vi "Benchmark SV Receive LV2012 - NI Verified - 1000 Byte - 1Var.vi"() -> ()   [LabVIEW 2019]
uses:
  <vilib>/Platform/TimedLoop/XDataNode/timing_clust.ctl
  <vilib>/Platform/TimedLoop/XDataNode/nitl_modes.ctl
  <vilib>/Platform/TimedLoop/XDataNode/wakeup.ctl
  <vilib>/platform/TimedLoop/XDataNode/XDataNode.xnode
  <vilib>/Platform/TimedLoop/XDataNode/XDNodeRunTimeDep.lvlib
panel:
  out "output cluster 2":T1
  in  "stop":bool
  in  "Server Closed":string="The server VI closed the connection."
  out "Time":u32
  out "Counter":i32
  # "Overview:  Coding that exemplifies how to benchmark the communication of Shared Variables.\nRequirements: LabVIEW 2012 or compatible\nInstructions:\n1. Run this VI\n2. Watch the amount of time it takes to communicate on the \"Benchmark SV Send  LV2012 - NI Verified.vi\" \n3. Stop both VIs"
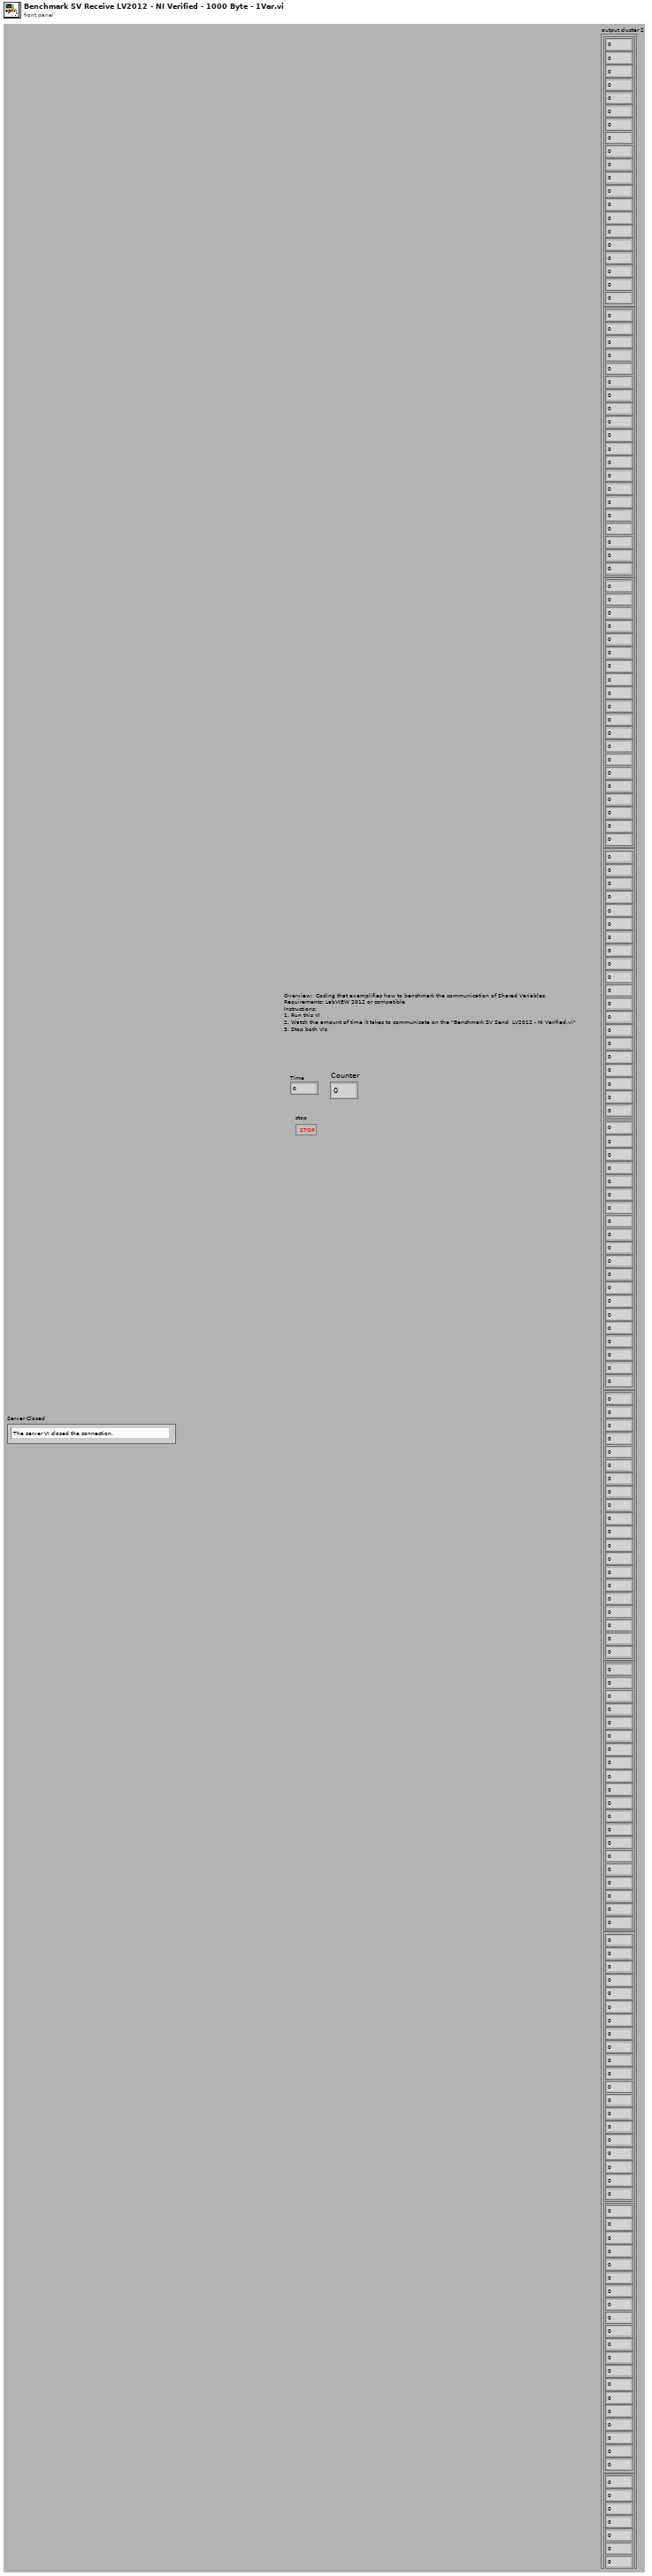
[diagram p1: front panel]
types:
  T1 = cluster{cluster{i64, i64, i64, i64, i64, i64, i64, i64, i64, i64, i64, i64, i64, i64, i64, i64, i64, i64, i64, i64}, cluster{i64, i64, i64, i64, i64, i64, i64, i64, i64, i64, i64, i64, i64, i64, i64, i64, i64, i64, i64, i64}, cluster{i64, i64, i64, i64, i64, i64, i64, i64, i64, i64, i64, i64, i64, i64, i64, i64, i64, i64, i64, i64}, cluster{i64, i64, i64, i64, i64, i64, i64, i64, i64, i64, i64, i64, i64, i64, i64, i64, i64, i64, i64, i64}, cluster{i64, i64, i64, i64, i64, i64, i64, i64, i64, i64, i64, i64, i64, i64, i64, i64, i64, i64, i64, i64}, cluster{i64, i64, i64, i64, i64, i64, i64, i64, i64, i64, i64, i64, i64, i64, i64, i64, i64, i64, i64, i64}, cluster{i64, i64, i64, i64, i64, i64, i64, i64, i64, i64, i64, i64, i64, i64, i64, i64, i64, i64, i64, i64}, cluster{i64, i64, i64, i64, i64, i64, i64, i64, i64, i64, i64, i64, i64, i64, i64, i64, i64, i64, i64, i64}, cluster{i64, i64, i64, i64, i64, i64, i64, i64, i64, i64, i64, i64, i64, i64, i64, i64, i64, i64, i64, i64}, cluster{i64, i64, i64, i64, i64, i64, i64, i64, i64, i64, i64, i64, i64, i64, i64, i64, i64, i64, i64, i64}, cluster{i64, i64, i64, i64, i64, i64, i64, i64, i64, i64, i64, i64, i64, i64, i64, i64, i64, i64, i64, i64}, cluster{i64, i64, i64, i64, i64, i64, i64, i64, i64, i64, i64, i64, i64, i64, i64, i64, i64, i64, i64, i64}, cluster{i64, i64, i64, i64, i64, i64, i64, i64, i64, i64, i64, i64, i64, i64, i64, i64, i64, i64, i64, i64}, cluster{i64, i64, i64, i64, i64, i64, i64, i64, i64, i64, i64, i64, i64, i64, i64, i64, i64, i64, i64, i64}, cluster{i64, i64, i64, i64, i64, i64, i64, i64, i64, i64, i64, i64, i64, i64, i64, i64, i64, i64, i64, i64}, cluster{i64, i64, i64, i64, i64, i64, i64, i64, i64, i64, i64, i64, i64, i64, i64, i64, i64, i64, i64, i64}, cluster{i64, i64, i64, i64, i64, i64, i64, i64, i64, i64, i64, i64, i64, i64, i64, i64, i64, i64, i64, i64}, cluster{i64, i64, i64, i64, i64, i64, i64, i64, i64, i64, i64, i64, i64, i64, i64, i64, i64, i64, i64, i64}, cluster{i64, i64, i64, i64, i64, i64, i64, i64, i64, i64, i64, i64, i64, i64, i64, i64, i64, i64, i64, i64}, cluster{i64, i64, i64, i64, i64, i64, i64, i64, i64, i64, i64, i64, i64, i64, i64, i64, i64, i64, i64, i64}, cluster{i64, i64, i64, i64, i64, i64, i64, i64, i64, i64, i64, i64, i64, i64, i64, i64, i64, i64, i64, i64}, cluster{i64, i64, i64, i64, i64, i64, i64, i64, i64, i64, i64, i64, i64, i64, i64, i64, i64, i64, i64, i64}, cluster{i64, i64, i64, i64, i64, i64, i64, i64, i64, i64, i64, i64, i64, i64, i64, i64, i64, i64, i64, i64}, cluster{i64, i64, i64, i64, i64, i64, i64, i64, i64, i64, i64, i64, i64, i64, i64, i64, i64, i64, i64, i64}, cluster{i64, i64, i64, i64, i64, i64, i64, i64, i64, i64, i64, i64, i64, i64, i64, i64, i64, i64, i64, i64}, cluster{i64, i64, i64, i64, i64, i64, i64, i64, i64, i64, i64, i64, i64, i64, i64, i64, i64, i64, i64, i64}, cluster{i64, i64, i64, i64, i64, i64, i64, i64, i64, i64, i64, i64, i64, i64, i64, i64, i64, i64, i64, i64}, cluster{i64, i64, i64, i64, i64, i64, i64, i64, i64, i64, i64, i64, i64, i64, i64, i64, i64, i64, i64, i64}, cluster{i64, i64, i64, i64, i64, i64, i64, i64, i64, i64, i64, i64, i64, i64, i64, i64, i64, i64, i64, i64}, cluster{i64, i64, i64, i64, i64, i64, i64, i64, i64, i64, i64, i64, i64, i64, i64, i64, i64, i64, i64, i64}, cluster{i64, i64, i64, i64, i64, i64, i64, i64, i64, i64, i64, i64, i64, i64, i64, i64, i64, i64, i64, i64}, cluster{i64, i64, i64, i64, i64, i64, i64, i64, i64, i64, i64, i64, i64, i64, i64, i64, i64, i64, i64, i64}, cluster{i64, i64, i64, i64, i64, i64, i64, i64, i64, i64, i64, i64, i64, i64, i64, i64, i64, i64, i64, i64}, cluster{i64, i64, i64, i64, i64, i64, i64, i64, i64, i64, i64, i64, i64, i64, i64, i64, i64, i64, i64, i64}, cluster{i64, i64, i64, i64, i64, i64, i64, i64, i64, i64, i64, i64, i64, i64, i64, i64, i64, i64, i64, i64}, cluster{i64, i64, i64, i64, i64, i64, i64, i64, i64, i64, i64, i64, i64, i64, i64, i64, i64, i64, i64, i64}, cluster{i64, i64, i64, i64, i64, i64, i64, i64, i64, i64, i64, i64, i64, i64, i64, i64, i64, i64, i64, i64}, cluster{i64, i64, i64, i64, i64, i64, i64, i64, i64, i64, i64, i64, i64, i64, i64, i64, i64, i64, i64, i64}, cluster{i64, i64, i64, i64, i64, i64, i64, i64, i64, i64, i64, i64, i64, i64, i64, i64, i64, i64, i64, i64}, cluster{i64, i64, i64, i64, i64, i64, i64, i64, i64, i64, i64, i64, i64, i64, i64, i64, i64, i64, i64, i64}, cluster{i64, i64, i64, i64, i64, i64, i64, i64, i64, i64, i64, i64, i64, i64, i64, i64, i64, i64, i64, i64}, cluster{i64, i64, i64, i64, i64, i64, i64, i64, i64, i64, i64, i64, i64, i64, i64, i64, i64, i64, i64, i64}, cluster{i64, i64, i64, i64, i64, i64, i64, i64, i64, i64, i64, i64, i64, i64, i64, i64, i64, i64, i64, i64}, cluster{i64, i64, i64, i64, i64, i64, i64, i64, i64, i64, i64, i64, i64, i64, i64, i64, i64, i64, i64, i64}, cluster{i64, i64, i64, i64, i64, i64, i64, i64, i64, i64, i64, i64, i64, i64, i64, i64, i64, i64, i64, i64}, cluster{i64, i64, i64, i64, i64, i64, i64, i64, i64, i64, i64, i64, i64, i64, i64, i64, i64, i64, i64, i64}, cluster{i64, i64, i64, i64, i64, i64, i64, i64, i64, i64, i64, i64, i64, i64, i64, i64, i64, i64, i64, i64}, cluster{i64, i64, i64, i64, i64, i64, i64, i64, i64, i64, i64, i64, i64, i64, i64, i64, i64, i64, i64, i64}, cluster{i64, i64, i64, i64, i64, i64, i64, i64, i64, i64, i64, i64, i64, i64, i64, i64, i64, i64, i64, i64}, cluster{i64, i64, i64, i64, i64, i64, i64, i64, i64, i64, i64, i64, i64, i64, i64, i64, i64, i64, i64, i64}}
  T2 = typedef "XDNodeRunTimeDep.lvlib/timing_clust.ctl" = cluster{"Expected End [f-1]":u64, "Actual End [f-1]":u64, "Finished Late? [f-1]":bool, "Expected End [i-1]":u64, "Actual End [i-1]":u64, "Finished Late? [i-1]":bool, "Expected Start [i]":u64, "Actual Start [i]":u64, "Expected Start [f]":u64, "Actual Start [f]":u64, "Source Name":string, "Structure Name":string, "Period":i64, "Deadline":i64, "Offset":i64, "Start":i64, "Priority":i32, "Timeout":i32, "Mode":T3, "Wakeup Reason":T4, "Error":errorcluster, "Source Type":string, "Secondary Source Type":string, "Global End Time":u64, "Global Start Time":u64, "Frame Duration":u64, "Iteration Duration":u64, "Assigned CPU":i32, "I/O Scan Engine Mode":u32}
  T3 = typedef "XDNodeRunTimeDep.lvlib/nitl_modes.ctl" = enum32{"No Change", "Process missed periods, maintain original phase", "Discard missed periods, maintain original phase", "Process missed periods, ignore original phase", "Discard missed periods, ignore original phase"}
  T4 = typedef "XDNodeRunTimeDep.lvlib/wakeup.ctl" = enum32{"Normal", "Aborted", "Asynchronous wakeup", "Timing source error", "Timed loop error", "Timeout"}
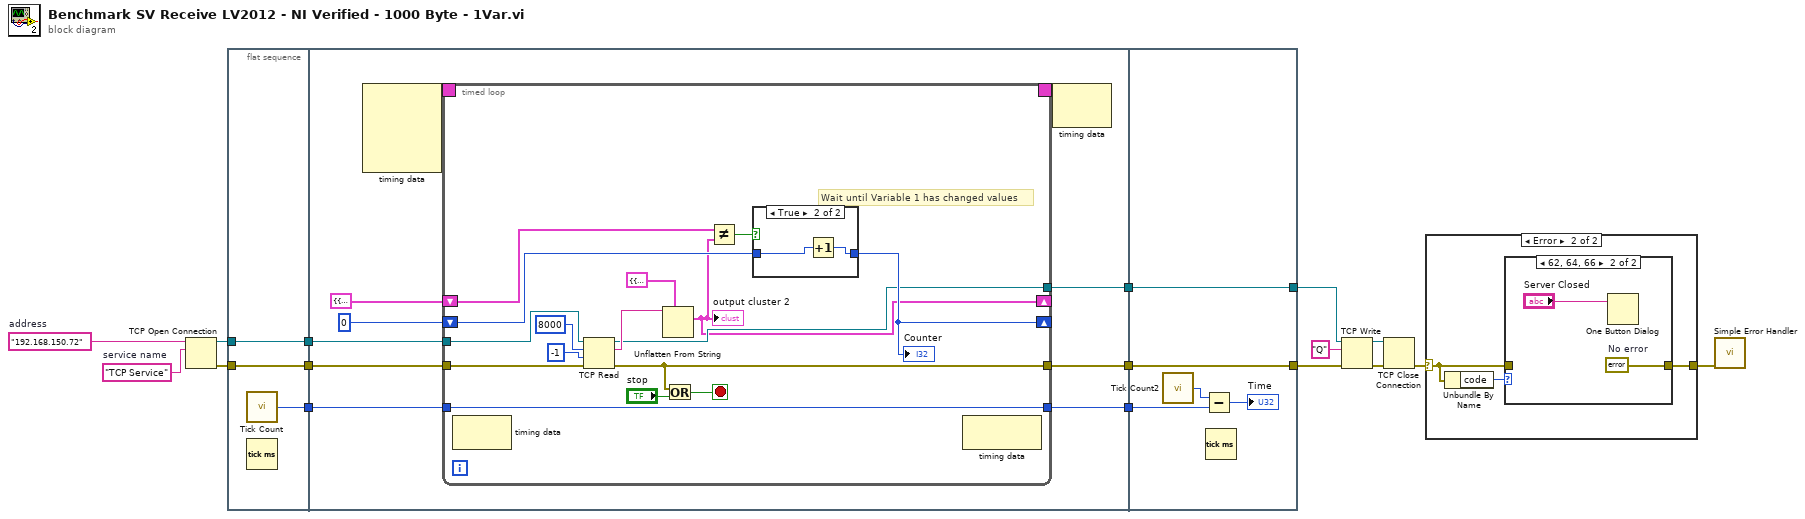
[diagram p0: block diagram]
diagram:
  w14 = "TCP Service"  # service name
  w1 = "192.168.150.72"  # address
  n1 = TCP Open Connection(address=w1, remote port or service name=w14) -> (connection ID=w13:refnum<k5>, error out=w12:errorcluster)  [unwired: 3 in]
  n2 = flat-sequence {
    tunnel: [w18] -> w17
    tunnel: w13 -> [w20]
    tunnel: w12 -> [w19]
    tunnel: [w20] -> w11
    tunnel: [w19] -> w10
    tunnel: [w29] -> w16
    tunnel: [w27] -> w15
    tunnel: w17 -> [w28]
    tunnel: w11 -> [w26]
    tunnel: w10 -> [w25]
    tunnel: [w24] -> w8
    tunnel: w16 -> [w56]
    tunnel: w15 -> [w57]
    tunnel: [w56] -> w7
    tunnel: [w55] -> w5
    tunnel: w8 -> [w55]
    frame #0 {
      n3 = call "Tick Count"() -> ("Tick Count(uSec)"=w18:u32)
      n4 = Tick Count (ms)() -> ()  [unwired: 1 out]
    }
    frame #1 {
      n5 = node-c288() -> (w23:T2)  [unwired: 4 in]
      n6 = timed-loop {
        shift-right: [w44] -> _
        shift-left: 0 -> [w46]
        tunnel: [w40] -> w27
        tunnel: w28 -> [w40]
        tunnel: w26 -> [w42]
        tunnel: [w38] -> w24
        shift-right: [w31] -> _
        shift-left: T1 {{0, 0, 0, 0, 0, 0, 0, 0, 0, 0, 0, 0, 0, 0, 0, 0, 0, 0, 0, 0}, {0, 0, 0, 0, 0, 0, 0, 0, 0, 0, 0, 0, 0, 0, 0, 0, 0, 0, 0, 0}, {0, 0, 0, 0, 0, 0, 0, 0, 0, 0, 0, 0, 0, 0, 0, 0, 0, 0, 0, 0}, {0, 0, 0, 0, 0, 0, 0, 0, 0, 0, 0, 0, 0, 0, 0, 0, 0, 0, 0, 0}, {0, 0, 0, 0, 0, 0, 0, 0, 0, 0, 0, 0, 0, 0, 0, 0, 0, 0, 0, 0}, {0, 0, 0, 0, 0, 0, 0, 0, 0, 0, 0, 0, 0, 0, 0, 0, 0, 0, 0, 0}, {0, 0, 0, 0, 0, 0, 0, 0, 0, 0, 0, 0, 0, 0, 0, 0, 0, 0, 0, 0}, {0, 0, 0, 0, 0, 0, 0, 0, 0, 0, 0, 0, 0, 0, 0, 0, 0, 0, 0, 0}, {0, 0, 0, 0, 0, 0, 0, 0, 0, 0, 0, 0, 0, 0, 0, 0, 0, 0, 0, 0}, {0, 0, 0, 0, 0, 0, 0, 0, 0, 0, 0, 0, 0, 0, 0, 0, 0, 0, 0, 0}, {0, 0, 0, 0, 0, 0, 0, 0, 0, 0, 0, 0, 0, 0, 0, 0, 0, 0, 0, 0}, {0, 0, 0, 0, 0, 0, 0, 0, 0, 0, 0, 0, 0, 0, 0, 0, 0, 0, 0, 0}, {0, 0, 0, 0, 0, 0, 0, 0, 0, 0, 0, 0, 0, 0, 0, 0, 0, 0, 0, 0}, {0, 0, 0, 0, 0, 0, 0, 0, 0, 0, 0, 0, 0, 0, 0, 0, 0, 0, 0, 0}, {0, 0, 0, 0, 0, 0, 0, 0, 0, 0, 0, 0, 0, 0, 0, 0, 0, 0, 0, 0}, {0, 0, 0, 0, 0, 0, 0, 0, 0, 0, 0, 0, 0, 0, 0, 0, 0, 0, 0, 0}, {0, 0, 0, 0, 0, 0, 0, 0, 0, 0, 0, 0, 0, 0, 0, 0, 0, 0, 0, 0}, {0, 0, 0, 0, 0, 0, 0, 0, 0, 0, 0, 0, 0, 0, 0, 0, 0, 0, 0, 0}, {0, 0, 0, 0, 0, 0, 0, 0, 0, 0, 0, 0, 0, 0, 0, 0, 0, 0, 0, 0}, {0, 0, 0, 0, 0, 0, 0, 0, 0, 0, 0, 0, 0, 0, 0, 0, 0, 0, 0, 0}, {0, 0, 0, 0, 0, 0, 0, 0, 0, 0, 0, 0, 0, 0, 0, 0, 0, 0, 0, 0}, {0, 0, 0, 0, 0, 0, 0, 0, 0, 0, 0, 0, 0, 0, 0, 0, 0, 0, 0, 0}, {0, 0, 0, 0, 0, 0, 0, 0, 0, 0, 0, 0, 0, 0, 0, 0, 0, 0, 0, 0}, {0, 0, 0, 0, 0, 0, 0, 0, 0, 0, 0, 0, 0, 0, 0, 0, 0, 0, 0, 0}, {0, 0, 0, 0, 0, 0, 0, 0, 0, 0, 0, 0, 0, 0, 0, 0, 0, 0, 0, 0}, {0, 0, 0, 0, 0, 0, 0, 0, 0, 0, 0, 0, 0, 0, 0, 0, 0, 0, 0, 0}, {0, 0, 0, 0, 0, 0, 0, 0, 0, 0, 0, 0, 0, 0, 0, 0, 0, 0, 0, 0}, {0, 0, 0, 0, 0, 0, 0, 0, 0, 0, 0, 0, 0, 0, 0, 0, 0, 0, 0, 0}, {0, 0, 0, 0, 0, 0, 0, 0, 0, 0, 0, 0, 0, 0, 0, 0, 0, 0, 0, 0}, {0, 0, 0, 0, 0, 0, 0, 0, 0, 0, 0, 0, 0, 0, 0, 0, 0, 0, 0, 0}, {0, 0, 0, 0, 0, 0, 0, 0, 0, 0, 0, 0, 0, 0, 0, 0, 0, 0, 0, 0}, {0, 0, 0, 0, 0, 0, 0, 0, 0, 0, 0, 0, 0, 0, 0, 0, 0, 0, 0, 0}, {0, 0, 0, 0, 0, 0, 0, 0, 0, 0, 0, 0, 0, 0, 0, 0, 0, 0, 0, 0}, {0, 0, 0, 0, 0, 0, 0, 0, 0, 0, 0, 0, 0, 0, 0, 0, 0, 0, 0, 0}, {0, 0, 0, 0, 0, 0, 0, 0, 0, 0, 0, 0, 0, 0, 0, 0, 0, 0, 0, 0}, {0, 0, 0, 0, 0, 0, 0, 0, 0, 0, 0, 0, 0, 0, 0, 0, 0, 0, 0, 0}, {0, 0, 0, 0, 0, 0, 0, 0, 0, 0, 0, 0, 0, 0, 0, 0, 0, 0, 0, 0}, {0, 0, 0, 0, 0, 0, 0, 0, 0, 0, 0, 0, 0, 0, 0, 0, 0, 0, 0, 0}, {0, 0, 0, 0, 0, 0, 0, 0, 0, 0, 0, 0, 0, 0, 0, 0, 0, 0, 0, 0}, {0, 0, 0, 0, 0, 0, 0, 0, 0, 0, 0, 0, 0, 0, 0, 0, 0, 0, 0, 0}, {0, 0, 0, 0, 0, 0, 0, 0, 0, 0, 0, 0, 0, 0, 0, 0, 0, 0, 0, 0}, {0, 0, 0, 0, 0, 0, 0, 0, 0, 0, 0, 0, 0, 0, 0, 0, 0, 0, 0, 0}, {0, 0, 0, 0, 0, 0, 0, 0, 0, 0, 0, 0, 0, 0, 0, 0, 0, 0, 0, 0}, {0, 0, 0, 0, 0, 0, 0, 0, 0, 0, 0, 0, 0, 0, 0, 0, 0, 0, 0, 0}, {0, 0, 0, 0, 0, 0, 0, 0, 0, 0, 0, 0, 0, 0, 0, 0, 0, 0, 0, 0}, {0, 0, 0, 0, 0, 0, 0, 0, 0, 0, 0, 0, 0, 0, 0, 0, 0, 0, 0, 0}, {0, 0, 0, 0, 0, 0, 0, 0, 0, 0, 0, 0, 0, 0, 0, 0, 0, 0, 0, 0}, {0, 0, 0, 0, 0, 0, 0, 0, 0, 0, 0, 0, 0, 0, 0, 0, 0, 0, 0, 0}, {0, 0, 0, 0, 0, 0, 0, 0, 0, 0, 0, 0, 0, 0, 0, 0, 0, 0, 0, 0}, {0, 0, 0, 0, 0, 0, 0, 0, 0, 0, 0, 0, 0, 0, 0, 0, 0, 0, 0, 0}} ("output cluster 2") -> [w37]
        tunnel: w25 -> [w43]
        tunnel: [w35] -> w29
        timing: w23 -> [_]
        timing-out: [_] -> w22
        stop <- w36 stop-if-true
        # "Wait until Variable 1 has changed values"
        n7 = node-c288() -> ()  [unwired: 1 in, 1 out]
        n8 = TCP Read(connection ID=w42, bytes to read=8000, error in (no error)=w43, 9:-1 ("timeout ms (25000)")) -> (connection ID out=w38:refnum<k5>, data out=w39:string, error out=w35:errorcluster)  [unwired: 1 in]
        n9 = Unflatten From String(type=T1 {{0, 0, 0, 0, 0, 0, 0, 0, 0, 0, 0, 0, 0, 0, 0, 0, 0, 0, 0, 0}, {0, 0, 0, 0, 0, 0, 0, 0, 0, 0, 0, 0, 0, 0, 0, 0, 0, 0, 0, 0}, {0, 0, 0, 0, 0, 0, 0, 0, 0, 0, 0, 0, 0, 0, 0, 0, 0, 0, 0, 0}, {0, 0, 0, 0, 0, 0, 0, 0, 0, 0, 0, 0, 0, 0, 0, 0, 0, 0, 0, 0}, {0, 0, 0, 0, 0, 0, 0, 0, 0, 0, 0, 0, 0, 0, 0, 0, 0, 0, 0, 0}, {0, 0, 0, 0, 0, 0, 0, 0, 0, 0, 0, 0, 0, 0, 0, 0, 0, 0, 0, 0}, {0, 0, 0, 0, 0, 0, 0, 0, 0, 0, 0, 0, 0, 0, 0, 0, 0, 0, 0, 0}, {0, 0, 0, 0, 0, 0, 0, 0, 0, 0, 0, 0, 0, 0, 0, 0, 0, 0, 0, 0}, {0, 0, 0, 0, 0, 0, 0, 0, 0, 0, 0, 0, 0, 0, 0, 0, 0, 0, 0, 0}, {0, 0, 0, 0, 0, 0, 0, 0, 0, 0, 0, 0, 0, 0, 0, 0, 0, 0, 0, 0}, {0, 0, 0, 0, 0, 0, 0, 0, 0, 0, 0, 0, 0, 0, 0, 0, 0, 0, 0, 0}, {0, 0, 0, 0, 0, 0, 0, 0, 0, 0, 0, 0, 0, 0, 0, 0, 0, 0, 0, 0}, {0, 0, 0, 0, 0, 0, 0, 0, 0, 0, 0, 0, 0, 0, 0, 0, 0, 0, 0, 0}, {0, 0, 0, 0, 0, 0, 0, 0, 0, 0, 0, 0, 0, 0, 0, 0, 0, 0, 0, 0}, {0, 0, 0, 0, 0, 0, 0, 0, 0, 0, 0, 0, 0, 0, 0, 0, 0, 0, 0, 0}, {0, 0, 0, 0, 0, 0, 0, 0, 0, 0, 0, 0, 0, 0, 0, 0, 0, 0, 0, 0}, {0, 0, 0, 0, 0, 0, 0, 0, 0, 0, 0, 0, 0, 0, 0, 0, 0, 0, 0, 0}, {0, 0, 0, 0, 0, 0, 0, 0, 0, 0, 0, 0, 0, 0, 0, 0, 0, 0, 0, 0}, {0, 0, 0, 0, 0, 0, 0, 0, 0, 0, 0, 0, 0, 0, 0, 0, 0, 0, 0, 0}, {0, 0, 0, 0, 0, 0, 0, 0, 0, 0, 0, 0, 0, 0, 0, 0, 0, 0, 0, 0}, {0, 0, 0, 0, 0, 0, 0, 0, 0, 0, 0, 0, 0, 0, 0, 0, 0, 0, 0, 0}, {0, 0, 0, 0, 0, 0, 0, 0, 0, 0, 0, 0, 0, 0, 0, 0, 0, 0, 0, 0}, {0, 0, 0, 0, 0, 0, 0, 0, 0, 0, 0, 0, 0, 0, 0, 0, 0, 0, 0, 0}, {0, 0, 0, 0, 0, 0, 0, 0, 0, 0, 0, 0, 0, 0, 0, 0, 0, 0, 0, 0}, {0, 0, 0, 0, 0, 0, 0, 0, 0, 0, 0, 0, 0, 0, 0, 0, 0, 0, 0, 0}, {0, 0, 0, 0, 0, 0, 0, 0, 0, 0, 0, 0, 0, 0, 0, 0, 0, 0, 0, 0}, {0, 0, 0, 0, 0, 0, 0, 0, 0, 0, 0, 0, 0, 0, 0, 0, 0, 0, 0, 0}, {0, 0, 0, 0, 0, 0, 0, 0, 0, 0, 0, 0, 0, 0, 0, 0, 0, 0, 0, 0}, {0, 0, 0, 0, 0, 0, 0, 0, 0, 0, 0, 0, 0, 0, 0, 0, 0, 0, 0, 0}, {0, 0, 0, 0, 0, 0, 0, 0, 0, 0, 0, 0, 0, 0, 0, 0, 0, 0, 0, 0}, {0, 0, 0, 0, 0, 0, 0, 0, 0, 0, 0, 0, 0, 0, 0, 0, 0, 0, 0, 0}, {0, 0, 0, 0, 0, 0, 0, 0, 0, 0, 0, 0, 0, 0, 0, 0, 0, 0, 0, 0}, {0, 0, 0, 0, 0, 0, 0, 0, 0, 0, 0, 0, 0, 0, 0, 0, 0, 0, 0, 0}, {0, 0, 0, 0, 0, 0, 0, 0, 0, 0, 0, 0, 0, 0, 0, 0, 0, 0, 0, 0}, {0, 0, 0, 0, 0, 0, 0, 0, 0, 0, 0, 0, 0, 0, 0, 0, 0, 0, 0, 0}, {0, 0, 0, 0, 0, 0, 0, 0, 0, 0, 0, 0, 0, 0, 0, 0, 0, 0, 0, 0}, {0, 0, 0, 0, 0, 0, 0, 0, 0, 0, 0, 0, 0, 0, 0, 0, 0, 0, 0, 0}, {0, 0, 0, 0, 0, 0, 0, 0, 0, 0, 0, 0, 0, 0, 0, 0, 0, 0, 0, 0}, {0, 0, 0, 0, 0, 0, 0, 0, 0, 0, 0, 0, 0, 0, 0, 0, 0, 0, 0, 0}, {0, 0, 0, 0, 0, 0, 0, 0, 0, 0, 0, 0, 0, 0, 0, 0, 0, 0, 0, 0}, {0, 0, 0, 0, 0, 0, 0, 0, 0, 0, 0, 0, 0, 0, 0, 0, 0, 0, 0, 0}, {0, 0, 0, 0, 0, 0, 0, 0, 0, 0, 0, 0, 0, 0, 0, 0, 0, 0, 0, 0}, {0, 0, 0, 0, 0, 0, 0, 0, 0, 0, 0, 0, 0, 0, 0, 0, 0, 0, 0, 0}, {0, 0, 0, 0, 0, 0, 0, 0, 0, 0, 0, 0, 0, 0, 0, 0, 0, 0, 0, 0}, {0, 0, 0, 0, 0, 0, 0, 0, 0, 0, 0, 0, 0, 0, 0, 0, 0, 0, 0, 0}, {0, 0, 0, 0, 0, 0, 0, 0, 0, 0, 0, 0, 0, 0, 0, 0, 0, 0, 0, 0}, {0, 0, 0, 0, 0, 0, 0, 0, 0, 0, 0, 0, 0, 0, 0, 0, 0, 0, 0, 0}, {0, 0, 0, 0, 0, 0, 0, 0, 0, 0, 0, 0, 0, 0, 0, 0, 0, 0, 0, 0}, {0, 0, 0, 0, 0, 0, 0, 0, 0, 0, 0, 0, 0, 0, 0, 0, 0, 0, 0, 0}, {0, 0, 0, 0, 0, 0, 0, 0, 0, 0, 0, 0, 0, 0, 0, 0, 0, 0, 0, 0}} ("output cluster 2"), binary string=w39) -> (value=w31:T1)  [unwired: 3 in, 2 out]
        "output cluster 2" <- w31
        n10 = Or(x=w35, y="stop") -> (x .or. y?=w36:bool)
        n11 = Not Equal?(x=w37, y=w31) -> (x != y?=w45:bool)
        n12 = case shown="True" w45 {
          tunnel: w46 -> [w49 w51]
          tunnel: [w49 w50] -> w44
          frame False {
          }
          frame True {
            n13 = Increment(x=w51) -> (x+1=w50:i32)
          }
        }
        "Counter" <- w44
        n14 = node-c288() -> ()  [unwired: 1 in, 1 out]
      }
      n15 = node-c288(w22) -> ()  [unwired: 1 out]
    }
    frame #2 {
      n16 = call "Tick Count2"() -> ("Tick Count(uSec)"=w54:u32)
      n17 = Subtract(x=w54, y=w57) -> (x-y=→"Time":u32)
      n18 = Tick Count (ms)() -> ()  [unwired: 1 out]
    }
  }
  n19 = TCP Write(connection ID=w5, data in="Q", error in (no error)=w7) -> (connection ID out=w2:refnum<k5>, error out=w4:errorcluster)  [unwired: 1 in, 1 out]
  n20 = TCP Close Connection(connection ID=w2, error in (no error)=w4) -> (error out=w3:errorcluster)  [unwired: 1 in, 1 out]
  n21 = case shown="Error" w3 {
    selector: w3 -> [w59 w61]
    tunnel: [w59 w60] -> w9
    frame No Error {
    }
    frame Error {
      n22 = Unbundle By Name(w61) -> ("code"=w62:i32)
      n23 = case shown="62, 64, 66" w62 {
        tunnel: w61 -> [w63 _]
        tunnel: [w63 w65] -> w60
        frame Default {
        }
        frame 62, 64, 66 {
          w65 = errorcluster {"status"=FALSE, "code"=0, "source"=""}  # No error
          n24 = One Button Dialog(message="Server Closed") -> ()  [unwired: 1 in, 1 out]
        }
      }
    }
  }
  n25 = call <vilib>:"Simple Error Handler.vi"("error in (no error)"=w9) -> ()  [unwired: 4 in, 5 out]
